vi "VI Server_GetLabels_Template.vi"() -> ()   [LabVIEW 2020, in "VI Server Toolkit LV2013.lvlib"]
doc: "Returns control labels of this VI except Labels - array which contains this labels.\nFor an example:\nYou need to create an array of control labels of your application which should be enabled/disabled for some reason. Instead of going from one control to another, just copy all of them into block diagram of this VI and run it. The Labels array will contain all other controls' labels."
uses:
  VI Server Toolkit LV2013.lvlib
panel:
  out "Labels":string[](array[string])
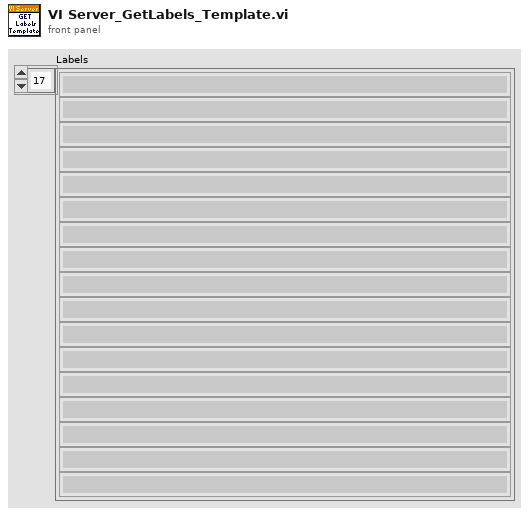
[diagram p1: front panel]
types:
  T1 = typedef "VI Server_RefsCluster.ctl" = cluster{"Labels":string[], "Refs":refnum<vi>[], "VI Ref":refnum<vi>}
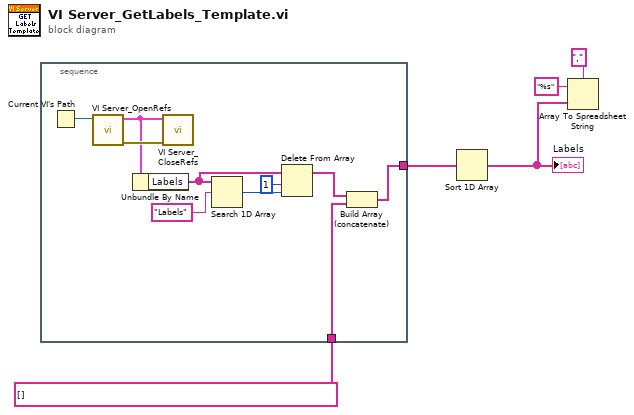
[diagram p0: block diagram]
diagram:
  n1 = stacked-sequence {
    tunnel: string[] [] -> [w7]
    tunnel: [w6] -> w4
    frame #0 {
      n2 = Current VI's Path() -> (path=w15:path)
      n3 = call "VI Server_OpenRefs.vi"("VI Path"=w15) -> ("error out"=w14:errorcluster, "VI Server.RefsCluster"=w13:T1)  [unwired: 9 in]
      n4 = Unbundle By Name(w13) -> ("Labels"=w9:string[])
      n5 = call "VI Server_CloseRefs.vi"("error in"=w14, "VI Server.RefsCluster"=w13) -> ()  [unwired: 9 in, 1 out]
      n6 = Search 1D Array(1D array=w9, element="Labels") -> (index of element=w10:i32)  [unwired: 1 in]
      n7 = Delete From Array(array=w9, length=1, index=w10) -> (array with subset deleted=w8:string[])  [unwired: 1 out]
      n8 = Build Array (concatenate)(w8, w7) -> (w6:string[])
    }
  }
  n9 = Sort 1D Array(array=w4) -> (sorted array=w3:string[])
  "Labels" <- w3
  n10 = Array To Spreadsheet String(delimiter (Tab)=",", array=w3, 3:"%s" ("format string")) -> ()  [unwired: 1 out]
